vi "Get Status.vi"() -> (2 "Command":string)   [LabVIEW 2017]
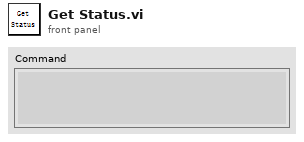
[diagram p1: front panel]
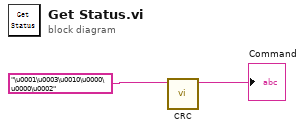
[diagram p0: block diagram]
diagram:
  n1 = call "CRC.vi"("字符串"="\u0001\u0003\u0010\u0000\u0000\u0002") -> ("连接的字符串"=→"Command":string)  [unwired: 9 in, 1 out]
